vi "Creat or Replace emibin.vi"(0 "file path":path, 5 "File type Std(0)":u8, 7 "File type ID":u16, 9 "File type Version":u8, 11 "error in (no error)":errorcluster) -> (4 "refnum out":refnum<file>, 15 "error out":errorcluster)   [LabVIEW 2011]
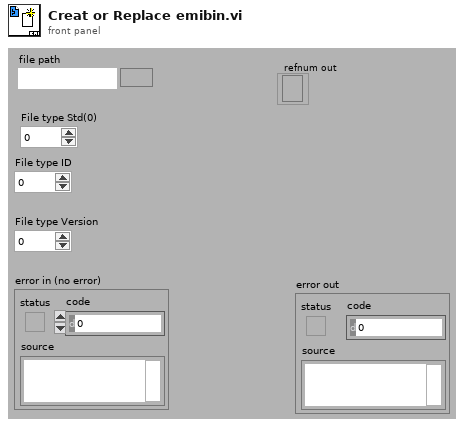
[diagram p1: front panel]
types:
  T1 = enum16{"big-endian, network order", "native, host order", "little-endian"}
  T2 = enum16{"open", "replace", "create", "open or create", "replace or create", "replace or create with confirmation"}
  T3 = typedef "Header.ctl" = cluster{"Fixed code":u32, "File type Std":u8, "File type ID":u16, "File type Version":u8}
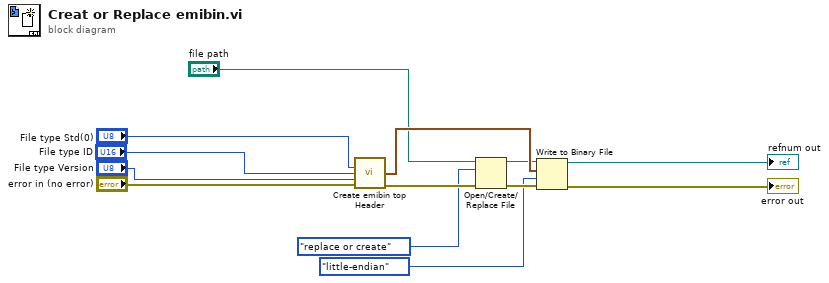
[diagram p0: block diagram]
diagram:
  n1 = call "Create emibin top Header.vi"("File type Std(0)"="File type Std(0)", "File type ID"="File type ID", "File type Version"="File type Version", "error in (no error)"="error in (no error)") -> ("bin ID header"=w8:T3, "error out"=w9:errorcluster)  [unwired: 10 in]
  n2 = Open/Create/Replace File(file path (use dialog)="file path", error in=w9, operation (0:open)=T2."replace or create") -> (refnum out=w4:refnum<file>, error out=w3:errorcluster)  [unwired: 3 in, 1 out]
  n3 = Write to Binary File(file (use dialog)=w4, data=w8, error in=w3, 9:T1."little-endian" ("byte order (0:big-endian, network order)")) -> (refnum out=→"refnum out":refnum<file>, error out=→"error out":errorcluster)  [unwired: 2 in, 1 out]
